vi "Set Current and Voltage.vi"(7 "Wait?":bool, 8 "error in (no error)":errorcluster, 9 "Current Limit":dbl, 10 "Voltage Limit":dbl, 11 "Magna Power in":refnum<class "Magna Power.lvclass">) -> (0 "error out":errorcluster, 3 "Magna Power out":refnum<class "Magna Power.lvclass">)   [LabVIEW 2015, in "Magna Power.lvclass"]
uses:
  Magna Power.lvclass
  Magna Power.lvclass/Magna Power.ctl
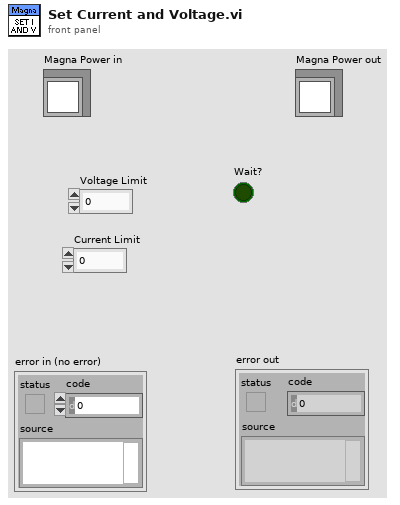
[diagram p1: front panel]
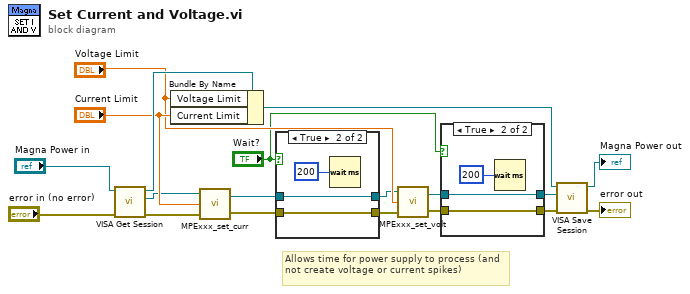
[diagram p0: block diagram]
diagram:
  # "Allows time for power supply to process (and not create voltage or current spikes)"
  n1 = call-dynamic "VISA Get Session.vi"("error in (no error)"="error in (no error)", "Instrument.lvclass in"="Magna Power in") -> ("error out"=w11:errorcluster, "VISA Resource Name"=w12:refnum<visa-resource-name>, "Instrument.lvclass out"=w18:refnum<class "Magna Power.lvclass">)  [unwired: 6 in, 1 out]
  n2 = Bundle By Name(cluster=w18, "Voltage Limit"="Voltage Limit", "Current Limit"="Current Limit") -> (w19:refnum<class "Magna Power.lvclass">)
  n3 = call "MPExxx_set_curr.vi"("error in (no error)"=w11, "Set Current"="Current Limit", "VISA session"=w12) -> ("error out"=w7:errorcluster, "dup VISA session"=w8:refnum<visa-resource-name>)
  n4 = case shown="True" "Wait?" {
    tunnel: [w21 w24] -> w9
    tunnel: w8 -> [w21 w24]
    tunnel: w7 -> [w20 w23]
    tunnel: [w20 w23] -> w6
    frame False {
    }
    frame True {
      n5 = Wait (ms)(milliseconds to wait=u32 200) -> ()  [unwired: 1 out]
    }
  }
  n6 = call "MPExxx_set_volt.vi"("error in (no error)"=w6, "Set Voltage"="Voltage Limit", "VISA session"=w9) -> ("error out"=w4:errorcluster, "dup VISA session"=w5:refnum<visa-resource-name>)
  n7 = case shown="True" "Wait?" {
    tunnel: [w26 w29] -> w2
    tunnel: w5 -> [w26 w29]
    tunnel: w4 -> [w25 w28]
    tunnel: [w25 w28] -> w3
    frame False {
    }
    frame True {
      n8 = Wait (ms)(milliseconds to wait=u32 200) -> ()  [unwired: 1 out]
    }
  }
  n9 = call-dynamic "VISA Save Session.vi"("error in (no error)"=w3, "VISA Resource Name"=w2, "Instrument.lvclass in"=w19) -> ("error out"=→"error out":errorcluster, "Instrument.lvclass out"=→"Magna Power out":refnum<class "Magna Power.lvclass">)  [unwired: 7 in]
